vi "flow rate names and values.vi"(10 "measurements":T1) -> (1 "values":dbl[](array[numeric]), 2 "names":string[](array[string]))   [LabVIEW 2013]
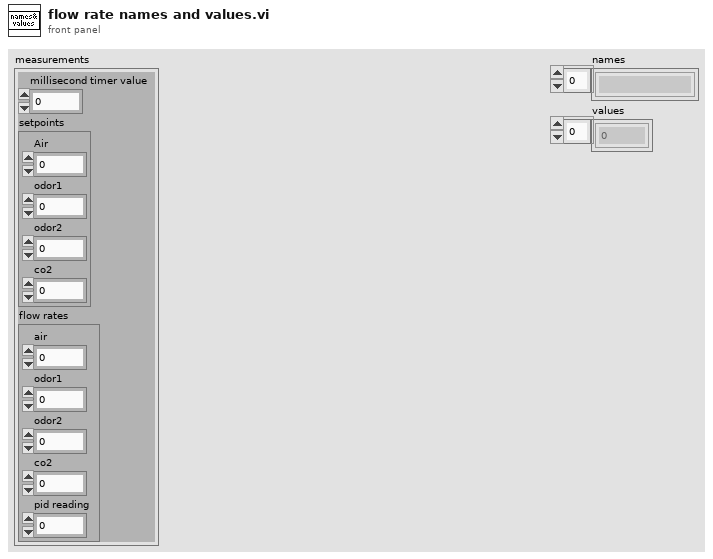
[diagram p1: front panel]
types:
  T1 = cluster{"millisecond timer value":u32, "setpoints ":cluster{"Air ":dbl, "odor1":dbl, "odor2":dbl, "co2":dbl}, "flow rates":cluster{"air":dbl, "odor1":dbl, "odor2":dbl, "co2":dbl, "pid reading":dbl}}
  T2 = cluster{"Air ":dbl, "odor1":dbl, "odor2":dbl, "co2":dbl}
  T3 = cluster{"air":dbl, "odor1":dbl, "odor2":dbl, "co2":dbl, "pid reading":dbl}
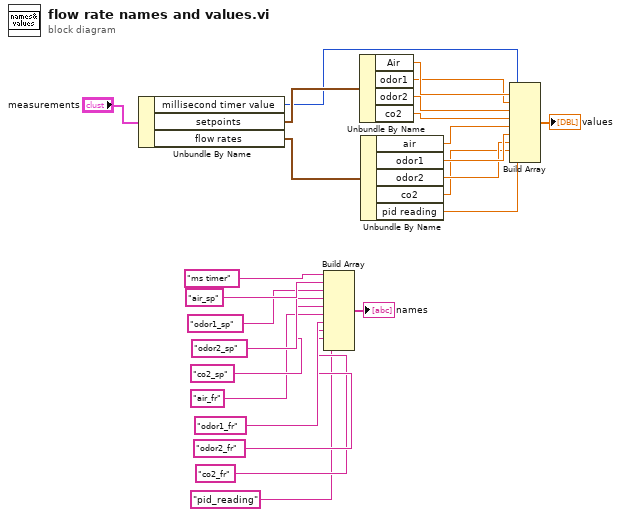
[diagram p0: block diagram]
diagram:
  n1 = Unbundle By Name("measurements") -> ("millisecond timer value"=w2:u32, "setpoints"=w24:T2, "flow rates"=w23:T3)
  n2 = Build Array("ms timer", "air_sp", "odor1_sp", "odor2_sp", "co2_sp", "air_fr", "odor1_fr", "odor2_fr", "co2_fr", "pid_reading") -> (→"names":string[])
  n3 = Unbundle By Name(w24) -> ("Air"=w11:dbl, "odor1"=w10:dbl, "odor2"=w9:dbl, "co2"=w8:dbl)
  n4 = Unbundle By Name(w23) -> ("air"=w7:dbl, "odor1"=w6:dbl, "odor2"=w5:dbl, "co2"=w4:dbl, "pid reading"=w3:dbl)
  n5 = Build Array(w2, w11, w10, w9, w8, w7, w6, w5, w4, w3) -> (→"values":dbl[])
